vi "对话框.vi"() -> ()   [LabVIEW 2018]
panel:
  out "字符串 2":string="您已经登录成功！！"
  out "密码 2":string caption="密码"
  out "用户名 2":string caption="用户名"
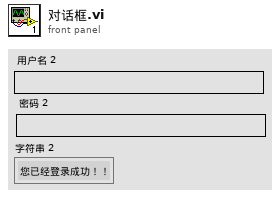
[diagram p1: front panel]
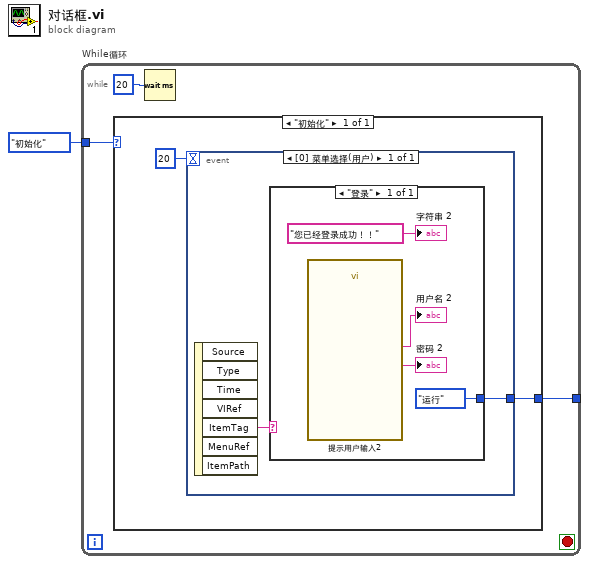
[diagram p0: block diagram]
diagram:
  n1 = while "While循环" {
    tunnel: enum16{"初始化"}."初始化" -> [w4]
    tunnel: [w2] -> _
    stop <- _ stop-if-true
    n2 = case shown="\"初始化\"" w4 {
      tunnel: [w5] -> w2
      frame "初始化" {
        n3 = event shown="[0] 菜单选择(用户)" {
          selector: _ -> [_]
          dyn-events: _ -> [_]
          timeout: 20 -> [_]
          tunnel: [w7] -> w5
          event Menu Selection (User) {
            n4 = event-data() -> ("ItemTag"=w8:string)  [unwired: 1 in, 6 out]
            n5 = case shown="\"登录\"" w8 {
              tunnel: [enum16{"运行"}."运行"] -> w7
              frame "登录" {
                n6 = call "提示用户输入2"() -> ("密码"=→"密码 2":string, "用户名"=→"用户名 2":string)  [unwired: 16 in, 2 out]
                "字符串 2" <- "您已经登录成功！！"
              }
            }
          }
        }
      }
    }
    n7 = Wait (ms)(milliseconds to wait=u32 20 ("等待时间（毫秒）")) -> ()  [unwired: 1 out]
  }
